vi "Configure Matching Circuit Embedding.vi"(0 "VISA resource name":refnum<visa-resource-name>, 1 "Circuit Mode (0: Normal)":u16(ring) items=["Normal", "Differential"], 2 "Circuit Type (0: None)":u16(ring) items=["None", "Series L Shunt C", "Shunt C Series L", "Shunt L Series C", "Series C Shunt L", "Shunt L Shunt C", "User"], 3 "C (0.0)":dbl format="%^.2e", 4 "G (0.0)":dbl format="%^.2e", 5 "error in (no error)":errorcluster, 6 "Channel (1)":i32=1, 7 "R (0.0)":dbl format="%^.2e", 8 "Port 1 (1)":i32=1, 9 "L (0.0)":dbl format="%^.2e", 10 "Matching State (F: Disable)":bool, 13 "File Name (\"\")":string) -> (14 "VISA resource name out":refnum<visa-resource-name>, 19 "error out":errorcluster)   [LabVIEW 2020, in "Agilent ENA Series.lvlib"]
doc: "Configures matching circuit embedding."
uses:
  <instrlib>/Agilent ENA Series/Agilent ENA Series.lvlib
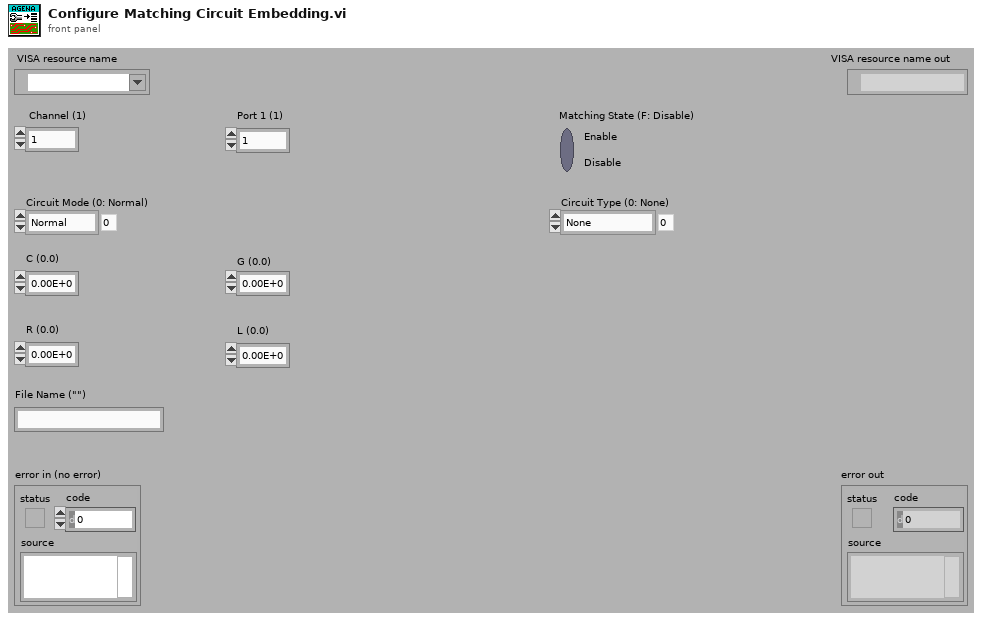
[diagram p1: front panel]
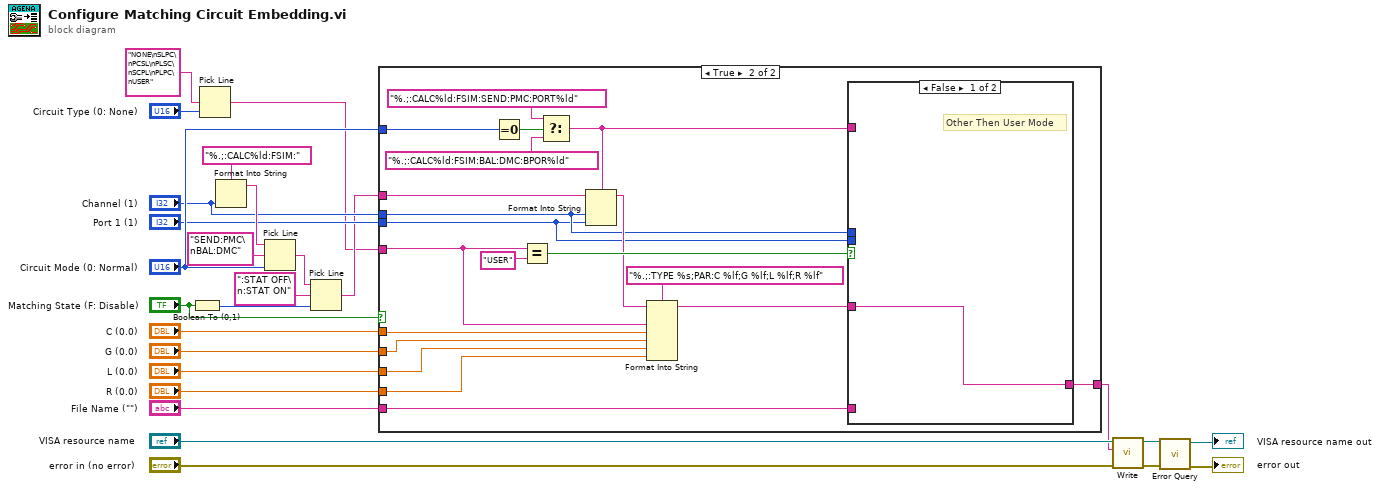
[diagram p0: block diagram]
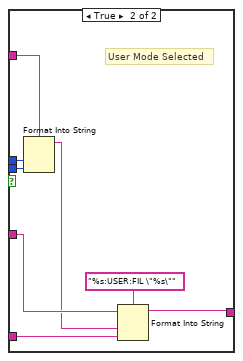
[diagram p3: hidden frame]
diagram:
  n1 = Boolean To (0,1)(Boolean="Matching State (F: Disable)") -> (0, 1=w20:i16)
  n2 = Pick Line(multi-line string="NONE\nSLPC\nPCSL\nPLSC\nSCPL\nPLPC\nUSER", line index="Circuit Type (0: None)") -> (output string=w11:string)  [unwired: 1 in]
  n3 = Format Into String(format string="%.;:CALC%ld:FSIM:", "Channel (1)") -> (resulting string=w22:string)  [unwired: 2 in, 1 out]
  n4 = Pick Line(string ("")=w22, multi-line string="SEND:PMC\nBAL:DMC", line index="Circuit Mode (0: Normal)") -> (output string=w19:string)
  n5 = Pick Line(string ("")=w19, multi-line string=":STAT OFF\n:STAT ON", line index=w20) -> (output string=w14:string)
  n6 = case shown="True" "Matching State (F: Disable)" {
    tunnel: "Circuit Mode (0: Normal)" -> [_ w45]
    tunnel: "Channel (1)" -> [_ w29]
    tunnel: "Port 1 (1)" -> [_ w28]
    tunnel: w14 -> [w27 w43]
    tunnel: w11 -> [_ w39]
    tunnel: "C (0.0)" -> [_ w38]
    tunnel: "G (0.0)" -> [_ w37]
    tunnel: "L (0.0)" -> [_ w36]
    tunnel: "R (0.0)" -> [_ w35]
    tunnel: [w27 w32] -> w5
    tunnel: "File Name (\"\")" -> [_ w34]
    frame False {
    }
    frame True {
      n7 = Equal To 0?(x=w45) -> (x = 0?=w44:bool)
      n8 = Equal?(x=w39, y="USER") -> (x = y?=w40:bool)
      n9 = Select(t="%.;:CALC%ld:FSIM:SEND:PMC:PORT%ld", s=w44, f="%.;:CALC%ld:FSIM:BAL:DMC:BPOR%ld" ("t")) -> (s? t:f=w30:string)
      n10 = Format Into String(format string=w30, initial string=w43, w29, w28) -> (resulting string=w31:string)  [unwired: 1 in, 1 out]
      n11 = Format Into String(format string="%.;:TYPE %s;PAR:C %lf;G %lf;L %lf;R %lf", initial string=w31, w39, w38, w37, w36, w35) -> (resulting string=w33:string)  [unwired: 1 in, 1 out]
      n12 = case shown="False" w40 {
        tunnel: w34 -> [_ w53]
        tunnel: [w48 w55] -> w32
        tunnel: w33 -> [w48 w54]
        tunnel: w30 -> [_ w52]
        tunnel: w29 -> [_ w50]
        tunnel: w28 -> [_ w49]
        frame False {
          # "Other Then User Mode"
        }
        frame True {
          # "User Mode Selected"
          n13 = Format Into String(format string=w52, w50, w49) -> (resulting string=w51:string)  [unwired: 2 in, 1 out]
          n14 = Format Into String(format string="%s:USER:FIL \"%s\"", initial string=w54, w51, w53) -> (resulting string=w55:string)  [unwired: 1 in, 1 out]
        }
      }
    }
  }
  n15 = call <instrlib>:"Write.vi"("error in (no error)"="error in (no error)", "String ()"=w5, "VISA resource name"="VISA resource name") -> ("error out"=w3:errorcluster, "VISA resource name out"=w4:refnum<visa-resource-name>)  [unwired: 6 in, 1 out]
  n16 = call <instrlib>:"Error Query.vi"("error in (no error)"=w3, "VISA resource name"=w4) -> ("error out"=→"error out":errorcluster, "VISA resource name out"=→"VISA resource name out":refnum<visa-resource-name>)  [unwired: 6 in, 2 out]
